vi "Shutdown.vi"(8 "error in (no error)":errorcluster, 9 "Params":variant, 11 "Module in":refnum<class "Module.lvclass">) -> (0 "error out":errorcluster, 3 "Module out":refnum<class "Module.lvclass">)   [LabVIEW 2020, in "Module.lvclass"]
uses:
  Module.lvclass
  controls/Request.ctl
  Get Module MQ.vi
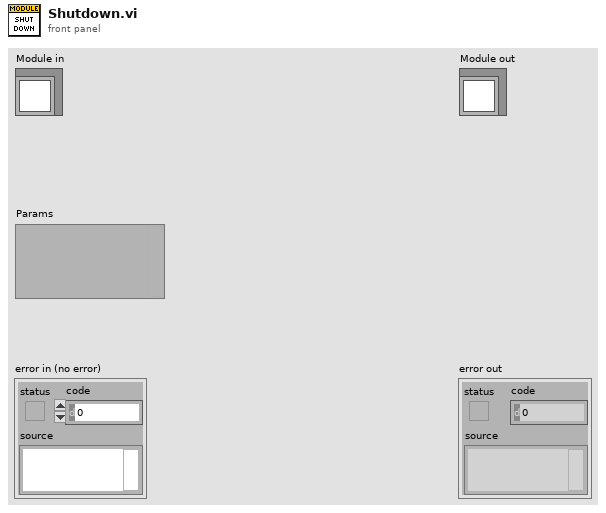
[diagram p1: front panel]
types:
  T1 = typedef "Request.ctl" = cluster{"Method":string, "Params":variant}
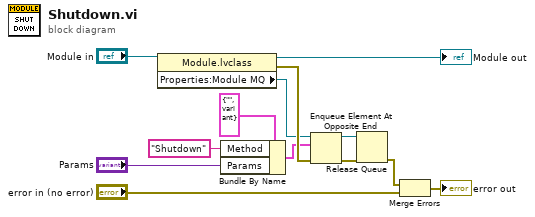
[diagram p0: block diagram]
diagram:
  n1 = property class="Module.lvclass"(reference="Module in") -> (reference out=→"Module out":refnum<class "Module.lvclass">, error out=w12:errorcluster, "Properties:Module MQ"=w11:refnum<queue>)  [unwired: 1 in]
  n2 = Bundle By Name(cluster=T1 {"Method"="", "Params"=variant} ("element"), "Method"="Shutdown" ("Message"), "Params"="Params") -> (w1:T1)
  n3 = Enqueue Element At Opposite End(queue=w11, element=w1, error in (no error)=w12) -> (queue out=w9:refnum<queue>, error out=w8:errorcluster)  [unwired: 1 in, 1 out]
  n4 = Release Queue(queue=w9, error in (no error)=w8) -> (error out=w7:errorcluster)  [unwired: 1 in, 2 out]
  n5 = Merge Errors(w7, "error in (no error)") -> (→"error out":errorcluster)
